vi "Actor Core.vi"(8 "error in":errorcluster, 11 "RootActor in":refnum<class "RootActor.lvclass">) -> (0 "error out":errorcluster, 3 "Actor out":refnum<class "Actor.lvclass">)   [LabVIEW 2020, in "RootActor.lvlib" / "RootActor.lvclass"]
doc: "(<B>Filename</B>: Actor Framework.lvlib:Actor.lvclass:Actor Core.vi)\n\nReceives messages to the actor, reacts to them, and initiates any error handling that may shut the actor down.\n\nDescendant classes may override this VI to append parallel tasks for the actor to complete while it handles messages. Overrides use the Call Parent Class Method node."
uses:
  RootActor.lvclass
  C:/Program Files (x86)/National Instruments/LabVIEW 2020/vi.lib/ActorFramework/Actor/Actor.lvclass
  <vilib>/ActorFramework/Actor/Actor.lvclass
  UI Status/UI Status/UI Status.lvclass
  RootActor.lvclass/RootActor.ctl
  <vilib>/ActorFramework/Actor/Actor.lvclass/Actor.ctl
  <vilib>/ActorFramework/Message Enqueuer/Message Enqueuer.lvclass/Message Enqueuer.ctl
  UI Status/UI Status Messages/Update Status Msg/Update Status Msg.lvclass/Update Status Msg.ctl
  <vilib>/ActorFramework/Message Enqueuer/Init from Existing Queue.vi
  <vilib>/ActorFramework/Message Enqueuer/Enqueue.vi
  <vilib>/ActorFramework/Stop Msg/Stop Msg.lvclass
  C:/Program Files (x86)/National Instruments/LabVIEW 2020/vi.lib/ActorFramework/Message/Message.lvclass
  UI Status/UI Status Messages/Update Status Msg/Update Status Msg.lvclass
  <vilib>/ActorFramework/Message Priority Queue/Priority Enqueue.vi
  <vilib>/ActorFramework/Message Enqueuer/Message Enqueuer.lvclass
panel:
  in  "Place Splitter":bool
  in  "OK Button":bool
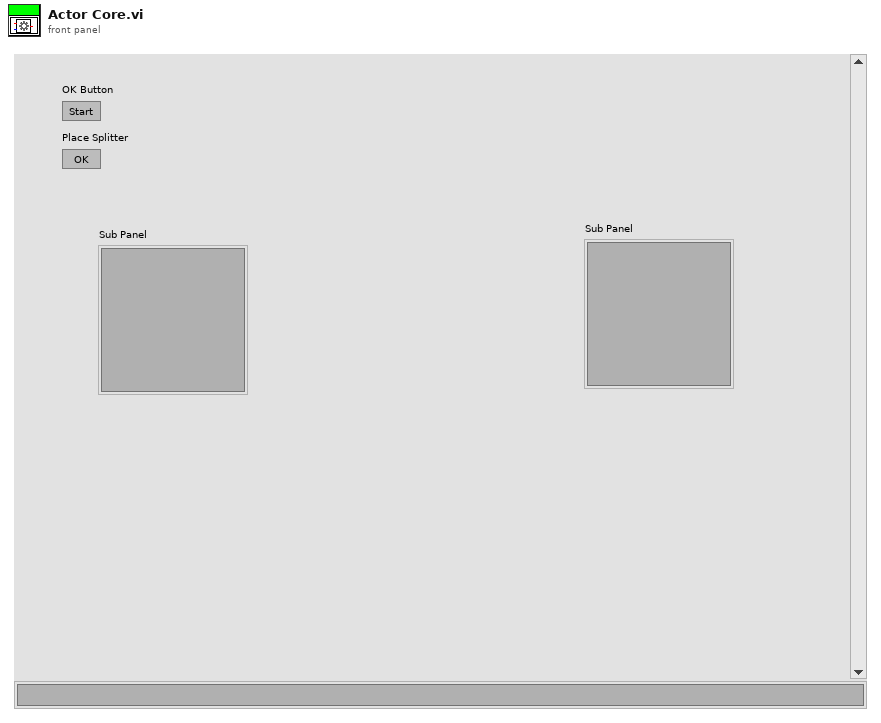
[diagram p1: front panel]
types:
  T1 = enum32{"Invalid", "Standard", "Closed", "Hidden", "Minimized", "Maximized"}
  T2 = cluster{"Stop":refnum<user-event>, "Clone Name":refnum<user-event>}
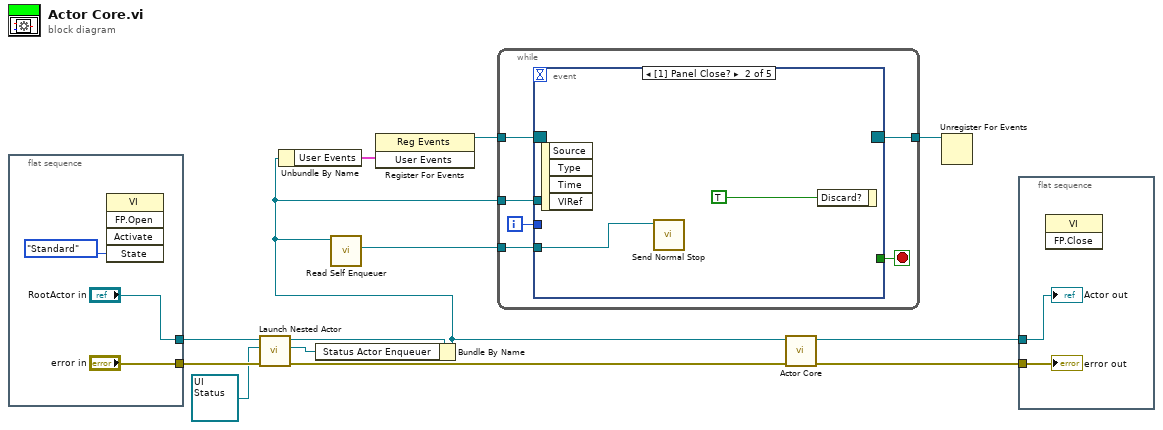
[diagram p0: block diagram]
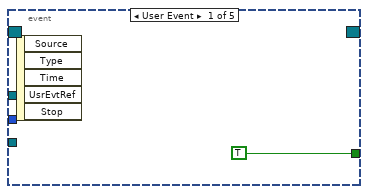
[diagram p2: hidden frame]
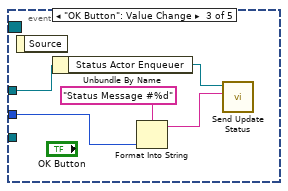
[diagram p3: hidden frame]
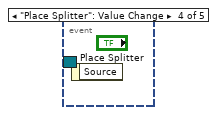
[diagram p4: hidden frame]
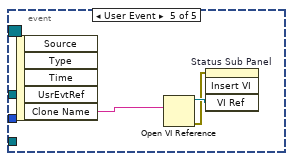
[diagram p5: hidden frame]
diagram:
  n1 = flat-sequence {
    tunnel: ["error in"] -> w7
    tunnel: ["RootActor in"] -> w2
    frame #0 {
      n2 = invoke class="VI" method="FP.Open"("State"=T1."Standard") -> ()  [unwired: 4 in, 5 out]
    }
  }
  n3 = call <vilib>:"Launch Nested Actor.vi"("error in (no error)"=w7, "Nested Actor"=refnum<class "UI Status.lvclass"> refnum ("UI Status.lvlib:UI Status.lvclass"), "Caller Actor in"=w2) -> ("error out"=w6:errorcluster, "Nested Actor's Enqueuer"=w3:refnum<class "Message Enqueuer.lvclass">, "Caller Actor out"=w4:refnum<class "RootActor.lvclass">)  [unwired: 6 in]
  n4 = Bundle By Name(cluster=w4, "Status Actor Enqueuer"=w3) -> (w1:refnum<class "RootActor.lvclass">)
  n5 = Unbundle By Name(w1) -> ("User Events"=w11:T2)
  n6 = call <vilib>:"Read Self Enqueuer.vi"("Actor"=w1) -> ("Self Enqueuer"=w8:refnum<class "Message Enqueuer.lvclass">)  [unwired: 10 in]
  n7 = register-events(w11) -> (reference out=w10:refnum<event-registration>)  [unwired: 2 in, 1 out]
  n8 = while {
    tunnel: w10 -> [w22]
    tunnel: [w20] -> w9
    tunnel: w8 -> [w19]
    tunnel: w1 -> [w18]
    i -> [w17]
    stop <- w21 stop-if-true
    n9 = event shown="[1] Panel Close?" {
      selector: w22 -> [_ _ _ _ _]
      dyn-events: [_ _ _ _ _] -> w20
      timeout: _ -> [_ _ _ _ _]
      tunnel: [TRUE _ _ _ _] -> w21
      tunnel: w19 -> [_ w24 _ _ _]
      tunnel: w18 -> [_ _ w30 _ _]
      tunnel: w17 -> [_ _ w28 _ _]
      event User Event {
        n10 = event-data() -> ()  [unwired: 1 in, 5 out]
      }
      event Panel Close? {
        n11 = event-data() -> ()  [unwired: 1 in, 4 out]
        n12 = call <vilib>:"Send Normal Stop.vi"("Message Enqueuer"=w24) -> ()  [unwired: 10 in, 1 out]
        n13 = event-data("Discard?"=TRUE) -> ()  [unwired: 1 in, 1 out]
      }
      event "OK Button": Value Change {
        n14 = event-data() -> ()  [unwired: 1 in, 1 out]
        n15 = Unbundle By Name(w30) -> ("Status Actor Enqueuer"=w29:refnum<class "Message Enqueuer.lvclass">)
        n16 = Format Into String(format string="Status Message #%d", w28) -> (resulting string=w26:string)  [unwired: 2 in, 1 out]
        n17 = call "Send Update Status.vi"("Status"=w26, "Message Enqueuer"=w29) -> ()  [unwired: 8 in, 2 out]
      }
      event "Place Splitter": Value Change {
        n18 = event-data() -> ()  [unwired: 1 in, 1 out]
      }
      event User Event {
        n19 = event-data() -> ("Clone Name"=w33:string)  [unwired: 1 in, 4 out]
        n20 = Open VI Reference(vi path=w33) -> (vi reference=w32:refnum<vi>, error out=w31:errorcluster)  [unwired: 5 in]
        n21 = invoke on="Status Sub Panel" class="SubPnl" method="Insert VI"(error in=w31, "VI Ref"=w32) -> ()  [unwired: 2 in, 4 out]
      }
    }
  }
  n22 = call-parent "Actor Core.vi"("error in"=w6, "Actor in"=w1) -> ("error out"=w13:errorcluster, "Actor out"=w12:refnum<class "Actor.lvclass">)  [unwired: 8 in]
  n23 = Unregister For Events(event registration refnum=w9) -> ()  [unwired: 1 in, 1 out]
  n24 = flat-sequence {
    tunnel: w13 -> [w35]
    tunnel: w12 -> [w34]
    frame #0 {
      n25 = invoke class="VI" method="FP.Close"() -> ()  [unwired: 3 in, 3 out]
      "error out" <- w35
      "Actor out" <- w34
    }
  }
